vi "PicoScope6000aNearestSampleIntervalStateless.vi"(5 "Enabled array":i16[](array[numeric])=[1, 0, 0, 0, 0, 0, 0, 0, 0, 0], 6 "Device Info":T1={"PICO_DRIVER_VERSION"="", "PICO_USB_VERSION"="", "PICO_HARDWARE_VERSION"="", "PICO_VARIANT_INFO"="", "PICO_BATCH_AND_SERIAL"="", "PICO_CAL_DATE"="", "PICO_KERNEL_VERSION"="", "PICO_DIGITAL_HARDWARE_VERSION"="", "PICO_ANALOGUE_HARDWARE_VERSION"="", "PICO_FIRMWARE_VERSION_1"="", "PICO_FIRMWARE_VERSION_2"="", "PICO_IPP_VERSION"="", "PICO_DRIVER_PATH"="", "PICO_FIRMWARE_VERSION_3"="", "PICO_FRONT_PANEL_FIRMWARE_VERSION"="", "Number of Channels"=4, "MSO"=FALSE}, 7 "Resolution":u32(ring)=10 items=["8-bit"=0, "12-bit"=1, "14-bit"=2, "15-bit"=3, "16-bit"=4, "10-bit"=10], 8 "error in (no error)":errorcluster, 9 "roundFaster":u8=1, 10 "timeIntervalRequested":dbl format="%#6_6p", 11 "handle in":i16) -> (0 "error out":errorcluster, 1 "timebase":u32, 2 "timeIntervalAvailable":dbl format="%#6_6p", 3 "handle out":i16)   [LabVIEW 2010]
doc: "Calls NearestSampleIntervalStateless function"
uses:
  ps6000a.dll
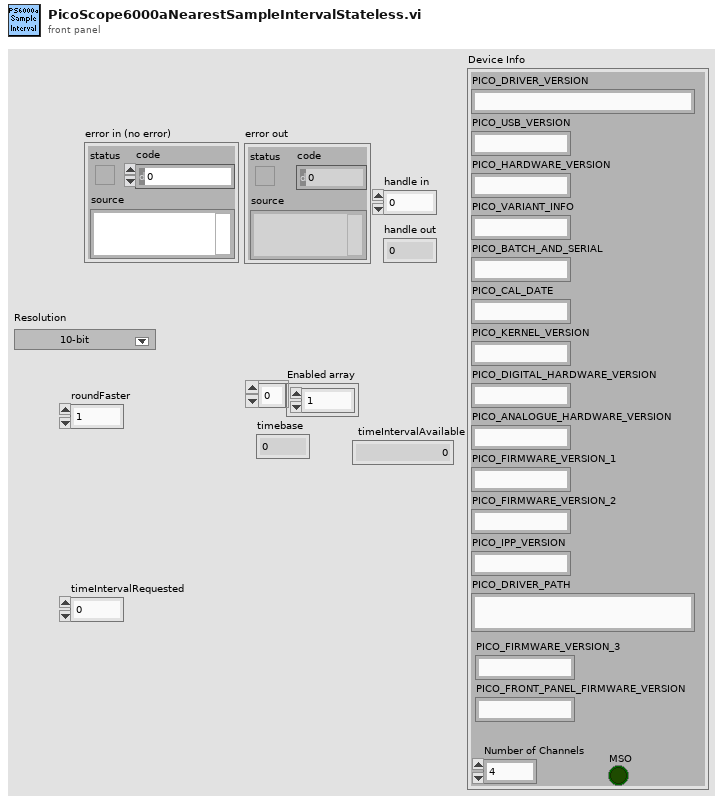
[diagram p1: front panel]
types:
  T1 = cluster{"PICO_DRIVER_VERSION":string, "PICO_USB_VERSION":string, "PICO_HARDWARE_VERSION":string, "PICO_VARIANT_INFO":string, "PICO_BATCH_AND_SERIAL":string, "PICO_CAL_DATE":string, "PICO_KERNEL_VERSION":string, "PICO_DIGITAL_HARDWARE_VERSION":string, "PICO_ANALOGUE_HARDWARE_VERSION":string, "PICO_FIRMWARE_VERSION_1":string, "PICO_FIRMWARE_VERSION_2":string, "PICO_IPP_VERSION":string, "PICO_DRIVER_PATH":string, "PICO_FIRMWARE_VERSION_3":string, "PICO_FRONT_PANEL_FIRMWARE_VERSION":string, "Number of Channels":i16, "MSO":bool}
  T2 = cluster{"status":bool, "code":u32, "source":string}
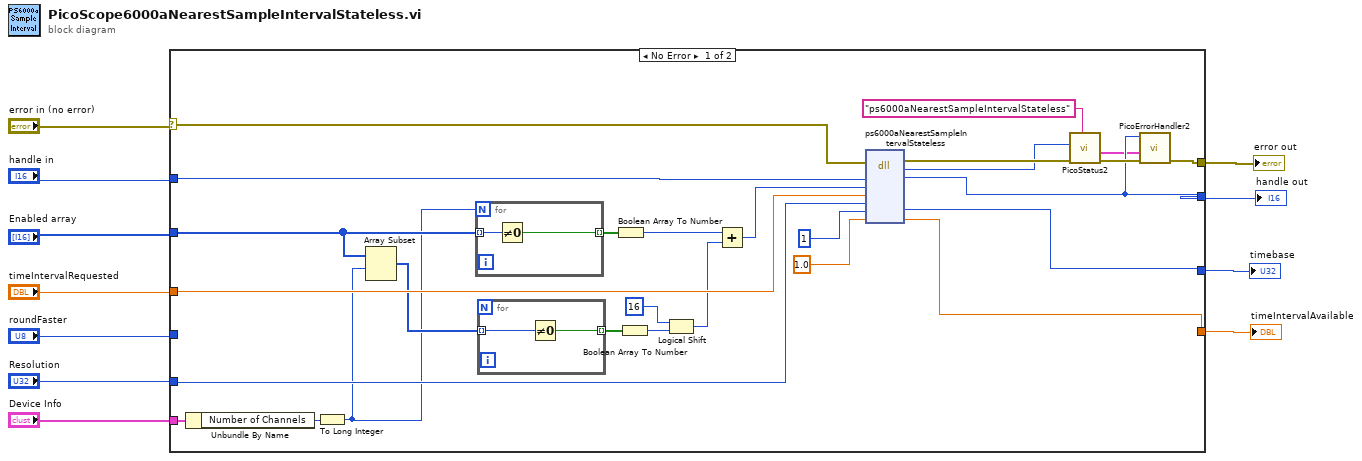
[diagram p0: block diagram]
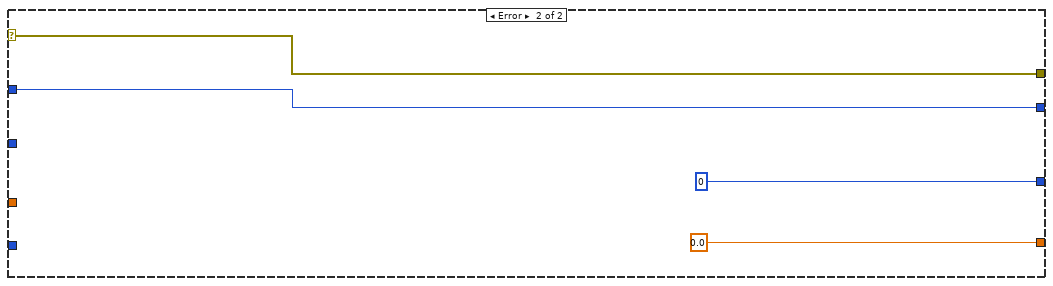
[diagram p2: hidden frame]
diagram:
  n1 = case shown="No Error" "error in (no error)" {
    selector: "error in (no error)" -> [w34 w46]
    tunnel: [w32 w46] -> w11
    tunnel: [w31 w45] -> w10
    tunnel: "handle in" -> [w35 w45]
    tunnel: "Enabled array" -> [w21 _]
    tunnel: "Resolution" -> [w27 _]
    tunnel: "roundFaster" -> [_ _]
    tunnel: "timeIntervalRequested" -> [w26 _]
    tunnel: [w25 u32 0 ("timebase")] -> w3
    tunnel: [w24 0.0 ("timeIntervalAvailable")] -> w2
    tunnel: "Device Info" -> [w22 _]
    frame No Error {
      n2 = Unbundle By Name(w22) -> ("Number of Channels"=w12:i16)
      n3 = To Long Integer(number=w12) -> (32bit integer=w13:i32)
      n4 = Array Subset(array=w21, index=w13) -> (w20:i16[])  [unwired: 1 in]
      n5 = for {
        N: w13 -> [_]
        tunnel: w21 -> [w42] mode=indexing
        tunnel: [w41] -> w28 mode=indexing
        n6 = Not Equal To 0?(x=w42) -> (x != 0?=w41:bool)
      }
      n7 = for {
        tunnel: w20 -> [w40] mode=indexing
        tunnel: [w39] -> w19 mode=indexing
        n8 = Not Equal To 0?(x=w40) -> (x != 0?=w39:bool)
      }
      n9 = Boolean Array To Number(Boolean array=w28) -> (number=w16:u32)
      n10 = Boolean Array To Number(Boolean array=w19) -> (number=w18:u32)
      n11 = Logical Shift(y=i16 16, x=w18) -> (x << y=w15:u32)
      n12 = Add(x=w16, y=w15) -> (x+y=w14:u32)
      n13 = dll-call lib="ps6000a.dll" fn="ps6000aNearestSampleIntervalStateless"(error in=w34, "handle"=w35, "enabledChannelFlags"=w14, "timeIntervalRequested"=w26, "resolution"=w27, "timebase"=u32 1, "timeIntervalAvailable"=1.0) -> (error out=w38:errorcluster, "PICO_STATUS"=w36:u32, "handle"=w31:i16, "timebase"=w25:u32, "timeIntervalAvailable"=w24:dbl)  [unwired: 5 in, 1 out]
      n14 = call "PicoStatus2.vi"("PICO source"="ps6000aNearestSampleIntervalStateless" ("source"), "Error in"=w38, "PICO STATUS"=w36) -> ("error out"=w33:errorcluster, "PICO_STATUS out"=w23:T2)  [unwired: 5 in]
      n15 = call "PicoErrorHandler2.vi"("error in (no error)"=w33, "PICO_STATUS in"=w23, "handle In"=w31) -> ("error out"=w32:errorcluster)  [unwired: 8 in]
    }
    frame Error {
    }
  }
  "error out" <- w11
  "handle out" <- w10
  "timebase" <- w3
  "timeIntervalAvailable" <- w2
